vi "查询一段时间数据sql.vi"(8 "结束时间":timestamp, 9 "起始时间":timestamp, 10 "表名":string, 11 "布尔":bool) -> (1 "error out":errorcluster, 3 "数据 2":string[][](array[string]))   [LabVIEW 2023]
panel:
  out "所得数据":variant[][](array[variant])
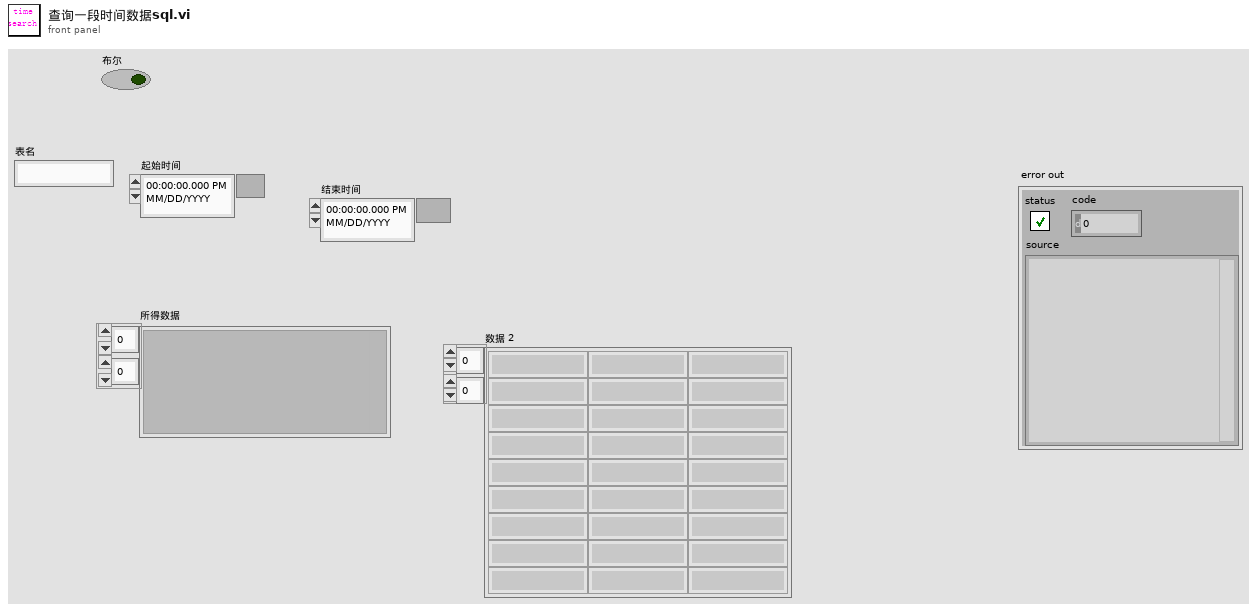
[diagram p1: front panel]
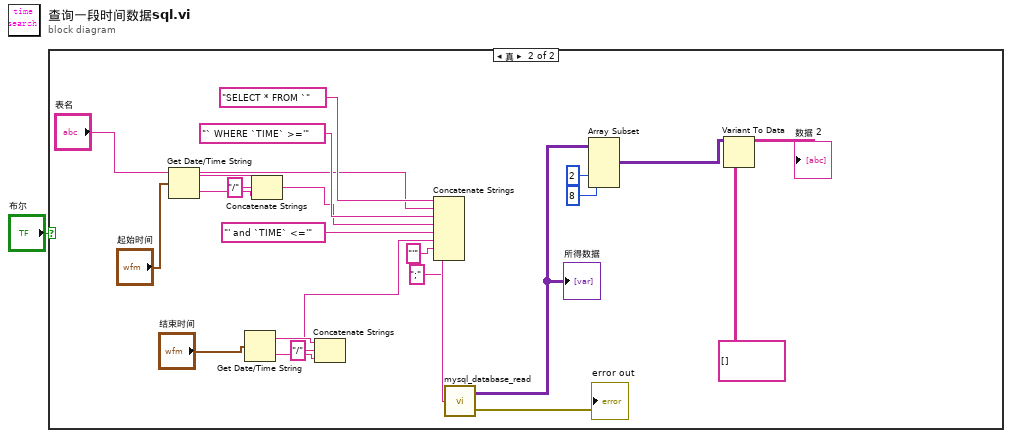
[diagram p0: block diagram]
diagram:
  n1 = case shown="真" "布尔" {
    frame False {
    }
    frame True {
      n2 = Get Date/Time String(seconds (now)="起始时间") -> (date string=w5:string, time string=w15:string)  [unwired: 2 in]
      n3 = Get Date/Time String(seconds (now)="结束时间") -> (date string=w13:string, time string=w3:string)  [unwired: 2 in]
      n4 = Concatenate Strings(w5, "/" ("字符串"), w15) -> (w14:string)
      n5 = Concatenate Strings(w13, "/" ("字符串"), w3) -> (w12:string)
      n6 = Concatenate Strings("SELECT * FROM `", "表名", "` WHERE `TIME` >='" ("字符串"), w14, "' and `TIME` <='" ("字符串"), w12, "'" ("数值文本.文本"), ";" ("字符串")) -> (w19:string)
      n7 = call "mysql_database_read.vi"("SQL query"=w19) -> ("recordset data"=w11:variant[][], "error out"=→"error out":errorcluster)
      "所得数据" <- w11
      n8 = Array Subset(array=w11, index (col)=2 ("索引"), length (col)=8 ("长度")) -> (w9:variant[][])  [unwired: 2 in]
      n9 = Variant To Data(type=string[][] [], Variant=w9) -> (data=→"数据 2":string[][])  [unwired: 1 in, 1 out]
    }
  }
